vi "Build Current Sense Section from XML.vi"(6 "Channels":refnum<k24>[](array[refnum]), 8 "error in (no error)":errorcluster, 9 "Card Position in":T1 {"Slot #" max=15}, 10 "Name in":string, 11 "Node Ptr in":u64) -> (0 "error out":errorcluster)   [LabVIEW 2014, in "SLSC configuration System Explorer.lvlib"]
uses:
  SLSC configuration System Explorer.lvlib
  Type Defs/Card Position.ctl
  Shared/SPI Utility/Slot #.ctl
  <vilib>/NI Veristand/Custom Device API/Custom Device Channel.ctl
  <vilib>/NI Veristand/Custom Device API/Custom Device Channel Type.ctl
  Shared/Constants.vi
  <vilib>/NI Veristand/Custom Device API/Custom Device API.lvlib
  Shared/SLSC configuration Shared.lvlib
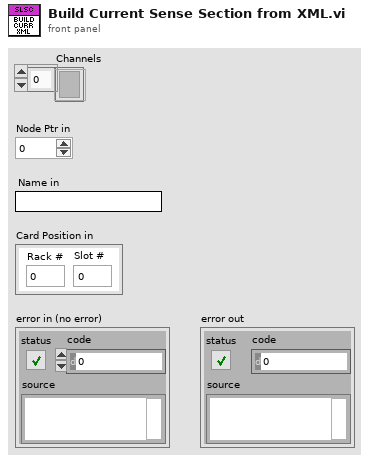
[diagram p1: front panel]
types:
  T1 = typedef "SLSC configuration Shared.lvlib/Card Position.ctl" = cluster{"Rack #":u8, "Slot #":T2}
  T2 = typedef "SLSC configuration Shared.lvlib/Slot #.ctl" = u8
  T3 = typedef "Custom Device API.lvlib/Custom Device Channel Type.ctl" = enum16{"Input", "Output"}
  T4 = typedef "Custom Device API.lvlib/Custom Device Channel.ctl" = cluster{"Type":T3, "Units":string, "Default Value":dbl, "Faultable":bool, "Scalable":bool}
  T5 = typedef "Custom Device API.lvlib/Custom Device Item Ref.ctl" = u64
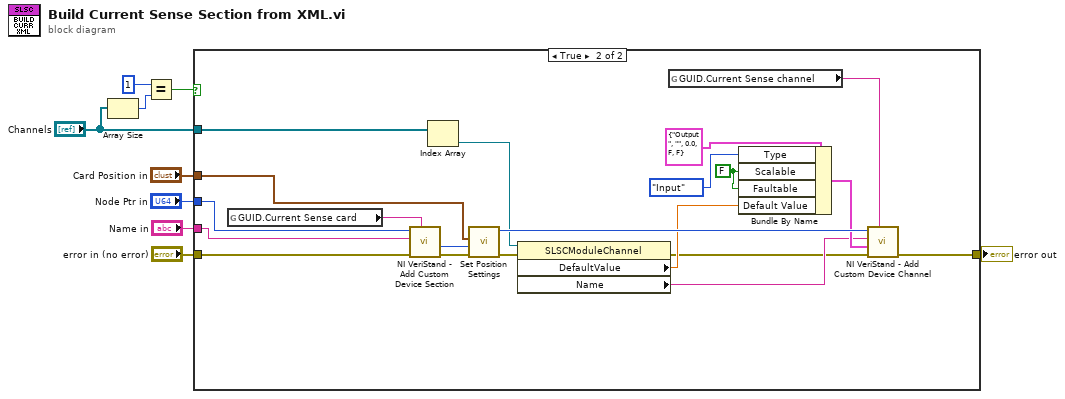
[diagram p0: block diagram]
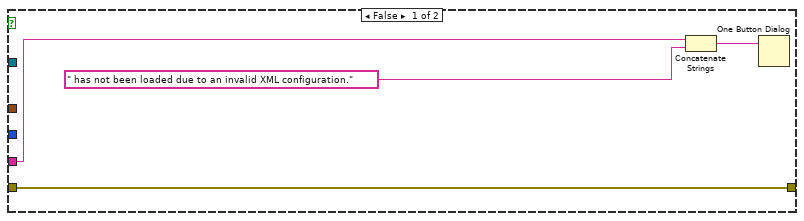
[diagram p2: hidden frame]
diagram:
  n1 = Array Size(array="Channels") -> (size(s)=w4:i32)
  n2 = Equal?(x=1, y=w4) -> (x = y?=w2:bool)
  n3 = case shown="True" w2 {
    tunnel: "error in (no error)" -> [w13 w33]
    tunnel: "Node Ptr in" -> [_ w32]
    tunnel: "Card Position in" -> [_ w29]
    tunnel: [w13 w16] -> w8
    tunnel: "Name in" -> [w10 w26]
    tunnel: "Channels" -> [_ w20]
    frame False {
      n4 = Concatenate Strings(w10, " has not been loaded due to an invalid XML configuration." ("string")) -> (w11:string)
      n5 = One Button Dialog(message=w11) -> ()  [unwired: 1 in, 1 out]
    }
    frame True {
      w22 = FALSE ("Scalable")
      n6 = global read "Constants.vi" "GUID.Current Sense card"() -> (w31:string)
      n7 = call <vilib>:"NI VeriStand - Add Custom Device Section.vi"("GUID (Default Section)"=w31, "error in (no error)"=w33, "Section Name"=w26, "Parent Ref in"=w32) -> ("error out"=w30:errorcluster, "Section Ptr"=w28:T5)  [unwired: 4 in, 2 out]
      n8 = Index Array(array=w20) -> (element=w18:refnum<k24>)  [unwired: 1 in]
      n9 = call "Set Position Settings.vi"("error in (no error)"=w30, "Card Position"=w29, "Item Ref in"=w28) -> ("error out"=w19:errorcluster, "Item Ref out"=w27:T5)  [unwired: 7 in]
      n10 = property class="SLSCModuleChannel"(reference=w18, error in=w19) -> (error out=w14:errorcluster, "DefaultValue"=w17:dbl, "Name"=w15:string)  [unwired: 1 out]
      n11 = global read "Constants.vi" "GUID.Current Sense channel"() -> (w21:string)
      n12 = Bundle By Name(cluster=T4 {"Type"=enum."Output", "Units"="", "Default Value"=0.0, "Faultable"=FALSE, "Scalable"=FALSE} ("Channel"), "Type"=Custom_Device_Channel_Type."Input", "Scalable"=w22, "Faultable"=w22, "Default Value"=w17) -> (w24:T4)
      n13 = call <vilib>:"NI VeriStand - Add Custom Device Channel.vi"("GUID (Default Channel)"=w21, "error in (no error)"=w14, "Channel"=w24, "Channel Name"=w15, "Parent Ref in"=w27) -> ("error out"=w16:errorcluster)  [unwired: 3 in, 3 out]
    }
  }
  "error out" <- w8
